vi "test.vi"() -> ()   [LabVIEW 2026]
panel:
  out "Waveform Graph":dbl[](graph)
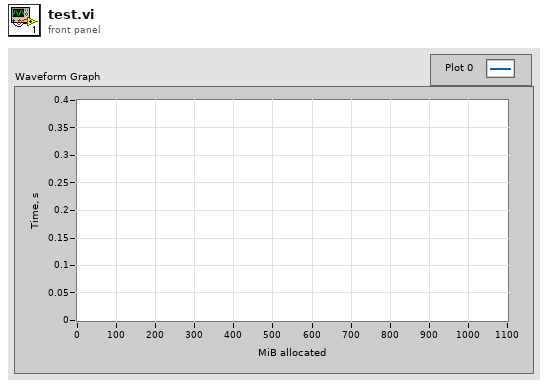
[diagram p1: front panel]
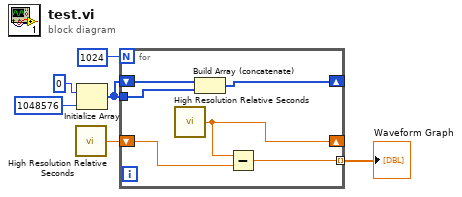
[diagram p0: block diagram]
diagram:
  n1 = call <vilib>:"High Resolution Relative Seconds.vi"() -> ("relative seconds"=w2:dbl)
  n2 = Initialize Array(u8 0 ("element"), 1048576 ("dimension size")) -> (w4:u8[])
  n3 = for {
    N: 1024 -> [_]
    shift-right: [w10] -> _
    shift-left: w4 -> [w12]
    tunnel: w4 -> [w11]
    shift-right: [w7] -> _
    shift-left: w2 -> [w9]
    tunnel: [w8] -> w1 mode=indexing
    n4 = call <vilib>:"High Resolution Relative Seconds.vi"() -> ("relative seconds"=w7:dbl)
    n5 = Build Array (concatenate)(w12, w11) -> (w10:u8[])
    n6 = Subtract(x=w7, y=w9) -> (x-y=w8:dbl)
  }
  "Waveform Graph" <- w1
